vi "Trigger subv ms based.vi"(0 "T=continuous, F=finite":bool, 2 "Initial delay [ms]":dbl=2.0 min=0.1 step=1.0, 3 "Pulse duration [ms]":dbl=2.0 min=0.1 step=1.0, 4 "Pulse frequency [Hz]":dbl=2.0 min=1.0 max=10000.0 step=1.0, 5 "Sample clock rate":dbl) -> (14 "ctr tasks out":refnum<k21>[](array[refnum]), 19 "error out":errorcluster)   [LabVIEW 2012]
doc: "SciScan 1.2 160622"
uses:
  <vilib>/DAQmx/create/channels.llb/DAQmx Create Channel (CO-Pulse Generation-Ticks).vi
  <vilib>/DAQmx/configure/timing.llb/DAQmx Timing (Implicit).vi
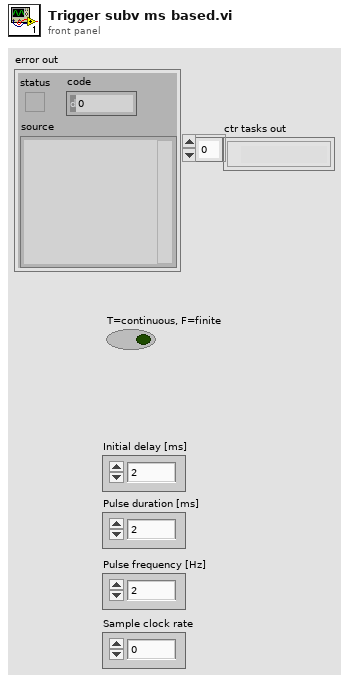
[diagram p1: front panel]
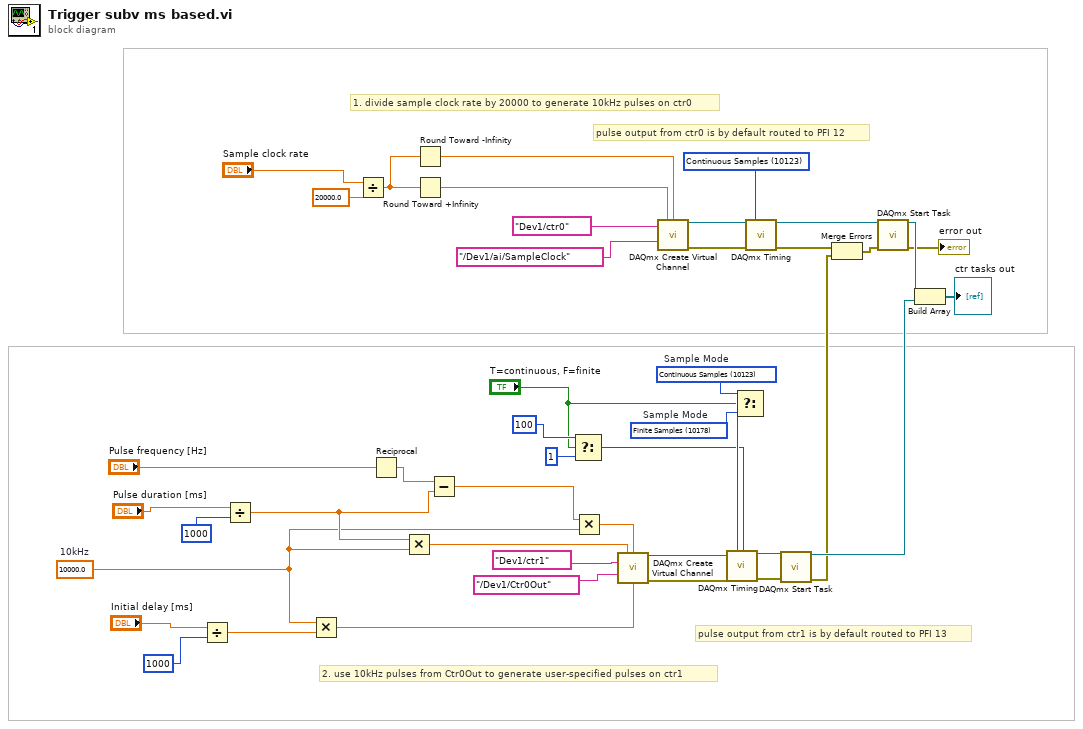
[diagram p0: block diagram]
diagram:
  w3 = 10123 items=["Finite Samples"=10178, "Continuous Samples"=10123, "Hardware Timed Single Point"=12522] ("sample mode")
  w12 = 10000.0  # 10kHz
  w28 = 10123 items=["Finite Samples"=10178, "Continuous Samples"=10123, "Hardware Timed Single Point"=12522]  # Sample Mode
  w29 = 10178 items=["Finite Samples"=10178, "Continuous Samples"=10123, "Hardware Timed Single Point"=12522]  # Sample Mode
  # "pulse output from ctr1 is by default routed to PFI 13"
  # "pulse output from ctr0 is by default routed to PFI 12"
  # "2. use 10kHz pulses from Ctr0Out to generate user-specified pulses on ctr1"
  # "1. divide sample clock rate by 20000 to generate 10kHz pulses on ctr0"
  n1 = Divide(x="Initial delay [ms]", y=1000) -> (x/y=w35:dbl)
  n2 = Divide(x="Pulse duration [ms]", y=1000) -> (x/y=w36:dbl)
  n3 = Multiply(x=w12, y=w35) -> (x*y=w33:dbl)
  n4 = Divide(x="Sample clock rate", y=20000.0 ("frequency")) -> (x/y=w15:dbl)
  n5 = Reciprocal(x="Pulse frequency [Hz]") -> (1/x=w38:dbl)
  n6 = Multiply(x=w36, y=w12) -> (x*y=w22:dbl)
  n7 = Round Toward -Infinity(1:w15) -> (0:w13:dbl)
  n8 = Round Toward +Infinity(x=w15) -> (ceil(x): smallest int >= x=w14:dbl)
  n9 = Subtract(x=w38, y=w36) -> (x-y=w37:dbl)
  n10 = Select(t=100, s="T=continuous, F=finite", f=1) -> (s? t:f=w26:i32)
  n11 = Multiply(x=w37, y=w12) -> (x*y=w21:dbl)
  n12 = call-poly <vilib>:"DAQmx Create Virtual Channel.vi"("high ticks"=w22, "low ticks"=w21, "counter"=tag "Dev1/ctr1", "source of ticks"=tag "/Dev1/Ctr0Out", "initial delay"=w33) -> ("task out"=w11:refnum<k21>, "error out"=w32:errorcluster)  [unwired: 9 in]
  n13 = call-poly <vilib>:"DAQmx Create Virtual Channel.vi"("high ticks"=w14, "low ticks"=w13, "counter"=tag "Dev1/ctr0", "source of ticks"=tag "/Dev1/ai/SampleClock") -> ("task out"=w19:refnum<k21>, "error out"=w20:errorcluster)  [unwired: 10 in]
  n14 = Select(t=w28, s="T=continuous, F=finite", f=w29) -> (s? t:f=w27:i32)
  n15 = call-poly <vilib>:"DAQmx Timing.vi"("task/channels in"=w11, "sample mode"=w27, "samples per channel"=w26, "error in"=w32) -> ("task out"=w30:refnum<k21>, "error out"=w31:errorcluster)  [unwired: 10 in]
  n16 = call-poly <vilib>:"DAQmx Timing.vi"("task/channels in"=w19, "sample mode"=w3, "error in"=w20) -> ("task out"=w8:refnum<k21>, "error out"=w7:errorcluster)  [unwired: 11 in]
  n17 = call <vilib>:"DAQmx Start Task.vi"("task/channels in"=w30, "error in"=w31) -> ("task out"=w23:refnum<k21>, "error out"=w1:errorcluster)  [unwired: 12 in]
  n18 = Merge Errors(w7, w1) -> (w6:errorcluster)
  n19 = call <vilib>:"DAQmx Start Task.vi"("task/channels in"=w8, "error in"=w6) -> ("task out"=w5:refnum<k21>, "error out"=→"error out":errorcluster)  [unwired: 12 in]
  n20 = Build Array(w5, w23) -> (→"ctr tasks out":refnum<k21>[])
